vi "Left Click.vi"(4 "Top  VI":refnum<vi>, 6 "Coords":T2, 7 "object refs":T1, 8 "error in (no error)":errorcluster, 9 "line name":string, 10 "Table Manager in":refnum<class "Table Manager.lvclass">, 11 "column in":refnum<class "Column.lvclass">) -> (0 "error out":errorcluster, 1 "Discard":bool, 2 "Table Manager out":refnum<class "Table Manager.lvclass">, 3 "column out":refnum<class "Column.lvclass">)   [LabVIEW 2013, in "Table Manager.lvlib" / "Column.lvclass"]
uses:
  Column.lvclass
  <vilib>/Utility/miscctls.llb/LVPoint32TypeDef.ctl
  Table Manager/object ref.ctl
  <vilib>/NI/DCAF/Tag Editor Core/Configuration Editor/Classes/Engine Parent/Engine Parent Editor Node.lvclass
  <vilib>/NI/DCAF/Tag Editor Core/Configuration Editor/Classes/Module editor node/module editor node.lvclass
  Table Manager/Table Manager.lvclass
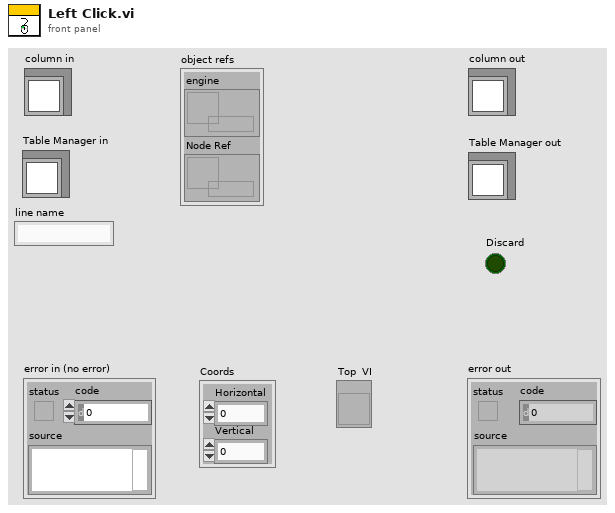
[diagram p1: front panel]
types:
  T1 = typedef "Table Manager.lvlib/Table Manager.lvclass/object ref.ctl" = cluster{"engine":refnum<data-value>, "Node Ref":refnum<data-value>}
  T2 = typedef "LVPoint32TypeDef.ctl" = cluster{"Horizontal":i32, "Vertical":i32}
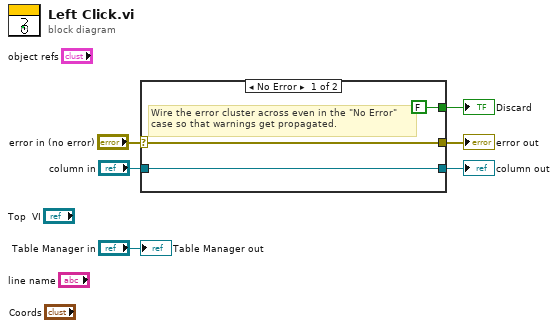
[diagram p0: block diagram]
diagram:
  n1 = case shown="No Error" "error in (no error)" {
    selector: "error in (no error)" -> [w8 w11]
    tunnel: [w8 w11] -> w5
    tunnel: [w9 w10] -> w3
    tunnel: "column in" -> [w9 w10]
    tunnel: [FALSE ("Discard") _] -> w2
    frame No Error {
      # "Wire the error cluster across even in the \"No Error\"\ncase so that warnings get propagated."
    }
    frame Error {
    }
  }
  "error out" <- w5
  "column out" <- w3
  "Discard" <- w2
  "Table Manager out" <- "Table Manager in"
